vi "InitChecklistCustom.vi"(1 "ListBox in":refnum<vi>) -> ()   [LabVIEW 2020]
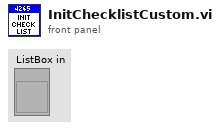
[diagram p1: front panel]
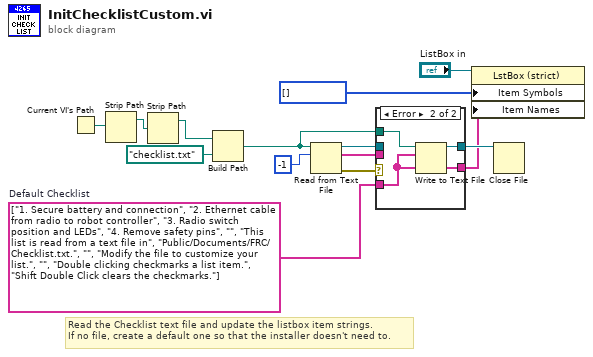
[diagram p0: block diagram]
diagram:
  w11 = string[] ["1. Secure battery and connection", "2. Ethernet cable from radio to robot controller", "3. Radio switch position and LEDs", "4. Remove safety pins", "", "This list is read from a text file in", "Public/Documents/FRC/Checklist.txt.", "", "Modify the file to customize your list.", "", "Double clicking checkmarks a list item.", "Shift Double Click clears the checkmarks."]  # Default Checklist
  # "Read the Checklist text file and update the listbox item strings.\nIf no file, create a default one so that the installer doesn't need to."
  n1 = Current VI's Path() -> (path=w4:path)
  n2 = Strip Path(path=w4) -> (stripped path=w3:path)  [unwired: 1 out]
  n3 = Strip Path(path=w3) -> (stripped path=w2:path)  [unwired: 1 out]
  n4 = Build Path(base path=w2, name or relative path=path "checklist.txt" ("XML File Path")) -> (appended path=w1:path)
  n5 = Read from Text File(file (use dialog)=w1, count=-1 ("timeout ms (25000)")) -> (refnum out=w13:refnum<file>, text=w10:string[], error out=w9:errorcluster)  [unwired: 2 in, 1 out]
  n6 = case shown="Error" w9 {
    tunnel: w10 -> [w16 _]
    tunnel: [w16 w18] -> w12
    tunnel: w11 -> [_ w18]
    tunnel: w1 -> [_ w19]
    tunnel: [w15 w17] -> w14
    tunnel: w13 -> [w15 _]
    frame No Error {
    }
    frame Error {
      n7 = Write to Text File(file (use dialog)=w19, text=w18) -> (refnum out=w17:refnum<file>)  [unwired: 2 in, 2 out]
    }
  }
  n8 = property on="Property Node" class="LstBox (strict)"(reference="ListBox in", "Item Symbols"=i32[] [], "Item Names"=w12) -> ()  [unwired: 1 in, 2 out]
  n9 = Close File(refnum=w14) -> ()  [unwired: 1 in, 2 out]
